vi "TestCompareCoords2.vi"() -> ()   [LabVIEW 2018]
panel:
  out "OUTPUT Z":dbl
  out "OUTPUT Y":dbl
  out "OUTPUT X":dbl
  out "INPUT Z":dbl=50.0
  out "INPUT X":dbl=260.0
  out "INPUT Y":dbl=-32.0
  in  "index":i32=17
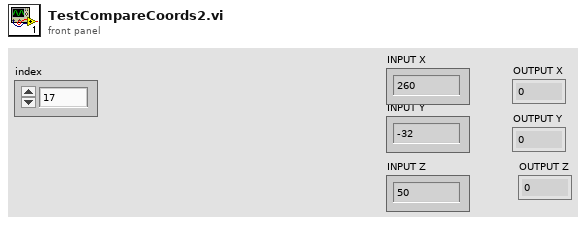
[diagram p1: front panel]
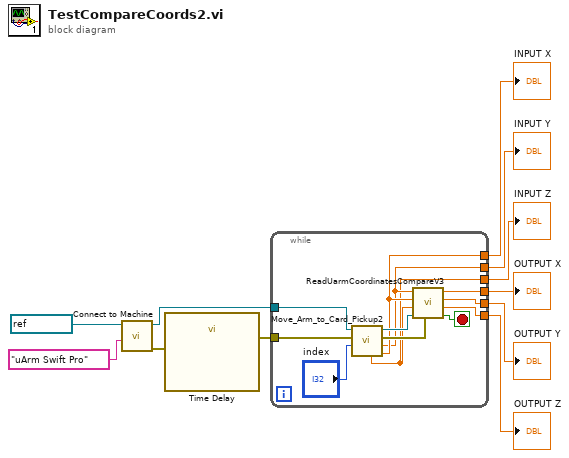
[diagram p0: block diagram]
diagram:
  n1 = call "Connect to Machine .vi"("Firmware"="uArm Swift Pro", "Machine In"=refnum<visa-resource-name> "COM6") -> ("error out"=w11:errorcluster, "Machine Out"=w8:refnum<visa-resource-name>)  [unwired: 7 in, 1 out]
  n2 = call "Time Delay"("error in (no error)"=w11) -> ("error out"=w7:errorcluster)  [unwired: 10 in]
  n3 = while {
    tunnel: w8 -> [w19]
    tunnel: w7 -> [w18]
    tunnel: [w23] -> w6
    tunnel: [w22] -> w5
    tunnel: [w21] -> w4
    tunnel: [w14] -> w3
    tunnel: [w13] -> w2
    tunnel: [w12] -> w1
    stop <- w20 stop-if-true
    n4 = call "Move_Arm_to_Card_Pickup2.vi"("index"="index", "error in"=w18, "Machine In"=w19) -> ("X Coordinate"=w14:dbl, "Y Coordinate"=w13:dbl, "error out"=w15:errorcluster, "Machine Out"=w16:refnum<visa-resource-name>, "Z Coordinate"=w12:dbl)  [unwired: 4 in]
    n5 = call "ReadUarmCoordinatesCompareV3.vi"("error out"=w15, "Machine Out"=w16, "INPUT Z Coord"=w12, "INPUT X Coord"=w14, "INPUT Y Coord"=w13) -> ("x = y?"=w20:bool, "OUTPUT Z Coord"=w21:dbl, "OUTPUT X Coord"=w22:dbl, "OUTPUT Y Coord"=w23:dbl)  [unwired: 3 in]
  }
  "INPUT Y" <- w2
  "INPUT X" <- w3
  "INPUT Z" <- w1
  "OUTPUT X" <- w6
  "OUTPUT Y" <- w5
  "OUTPUT Z" <- w4
